vi "Stop Core.vi"(10 "final error code":i32, 11 "ParentActor in":refnum<class "ParentActor.lvclass">) -> (3 "ParentActor out":refnum<class "ParentActor.lvclass">)   [LabVIEW 2020, in "ParentActor.lvclass"]
doc: "(<B>Filename</B>: Actor Framework.lvlib:Actor.lvclass:Stop Core.vi)\n\nDefines what the actor does before it stops. Use the <B>final error code</B> input to determine whether the actor shut down in response to an error.\n\nBy default, this method passes the Stop message along to all auto-stop nested actors. A descendant class may override this method to define additional behavior, such as shutting down any processes the actor initiated in its override of the Actor Core method."
uses:
  ParentActor/ParentActor.lvclass
  ParentActor/ParentActor.lvclass/ParentActor.ctl
  <vilib>/ActorFramework/Actor/Actor.lvclass
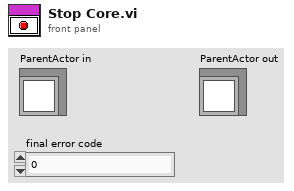
[diagram p1: front panel]
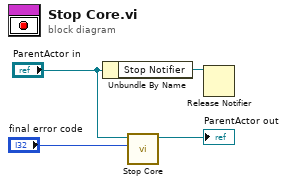
[diagram p0: block diagram]
diagram:
  n1 = Unbundle By Name("ParentActor in") -> ("Stop Notifier"=w1:refnum<notifier>)
  n2 = call-parent "Stop Core.vi"("final error code"="final error code", "Actor in"="ParentActor in") -> ("Actor out"=→"ParentActor out":refnum<class "ParentActor.lvclass">)  [unwired: 9 in]
  n3 = Release Notifier(notifier=w1) -> ()  [unwired: 2 in, 3 out]
